vi "simulation.vi"(1 "Stop signaller":refnum<class "Signaller.lvclass">, 2 "Frequency refnum":refnum<vi>, 3 "Data input file refnum":refnum<vi>) -> ()   [LabVIEW 2015]
uses:
  Fit Parameters.ctl
  Physical Constants.ctl
  Internal Parameters.ctl
  System parameters.ctl
  Motor controller/Signaller/Signaller.lvclass
  <vilib>/Platform/TimedLoop/XDataNode/timing_clust.ctl
  <vilib>/Platform/TimedLoop/XDataNode/nitl_modes.ctl
  <vilib>/Platform/TimedLoop/XDataNode/wakeup.ctl
  <vilib>/Platform/TimedLoop/scheduler/LVUserAPI/_suppVIs/Create_1kHz_TSource.vi
  <vilib>/Utility/file.llb/Write Delimited Spreadsheet (string).vi
  <vilib>/platform/TimedLoop/XDataNode/XDataNode.xnode
  <vilib>/Platform/TimedLoop/XDataNode/XDNodeRunTimeDep.lvlib
panel:
  in  "Precision":i32=100 min=1
  in  "Reset simulation":bool
  in  "Paused":bool=TRUE
  out "Current time (simulated)":timestamp format="%<%H:%M:%S\n%B %d, %Y>T"
  in  "Stop simulation":bool
  in  "Data output file":path
  out "Polarization":dbl
  in  "Beam on":bool
  in  "Time per second (s)":dbl=1.0
  out "Seconds until next data":u32
  in  "# Sweeps":u32=250
  out "Fit parameters chooser":refnum<vi>
  in  "Sweep error":dbl=0.01 min=0.0 format="%#_13g"
  out "Start time":timestamp
  out "Polarization (unfuzzed)":dbl
  in  "Thermal fluctuations":dbl=0.01 min=0.0
  out "Pn (noisy)":dbl
  in  "System parameters":T1={"Frequency"=140.2, "System temperature"=1.0, "Beam current"=100.0}
  out "Internal parameters":T2={"Pe"=-1.0, "Pn"=0.0, "Alpha"=0.0, "Beta"=0.0, "C"=0.000136073, "Phi"=0.0, "Pe0"=-1.0, "Dose"=0.0, "Temperature"=1.0}
  in  "Physical constants":T3={"T1e (s)"=0.03, "T1n (s)"=1500.0}
  in  "Fit parameters":T4={"A"=0.572086, "S"=0.0835606, "M1"=140.286, "M2"=140.486}
  in  "Launch fit parameters chooser":bool
  out "Elapsed time (s)":dbl
  in  "Add 30 minutes":bool
  in  "30 minutes":bool
  in  "15 minutes":bool
  in  "5 minutes":bool
  in  "Time scale (min)":i64=5 min=1
  out "Polarization vs time":cluster{timestamp[], dbl[]}(graph)
  # "Advanced data and controls"
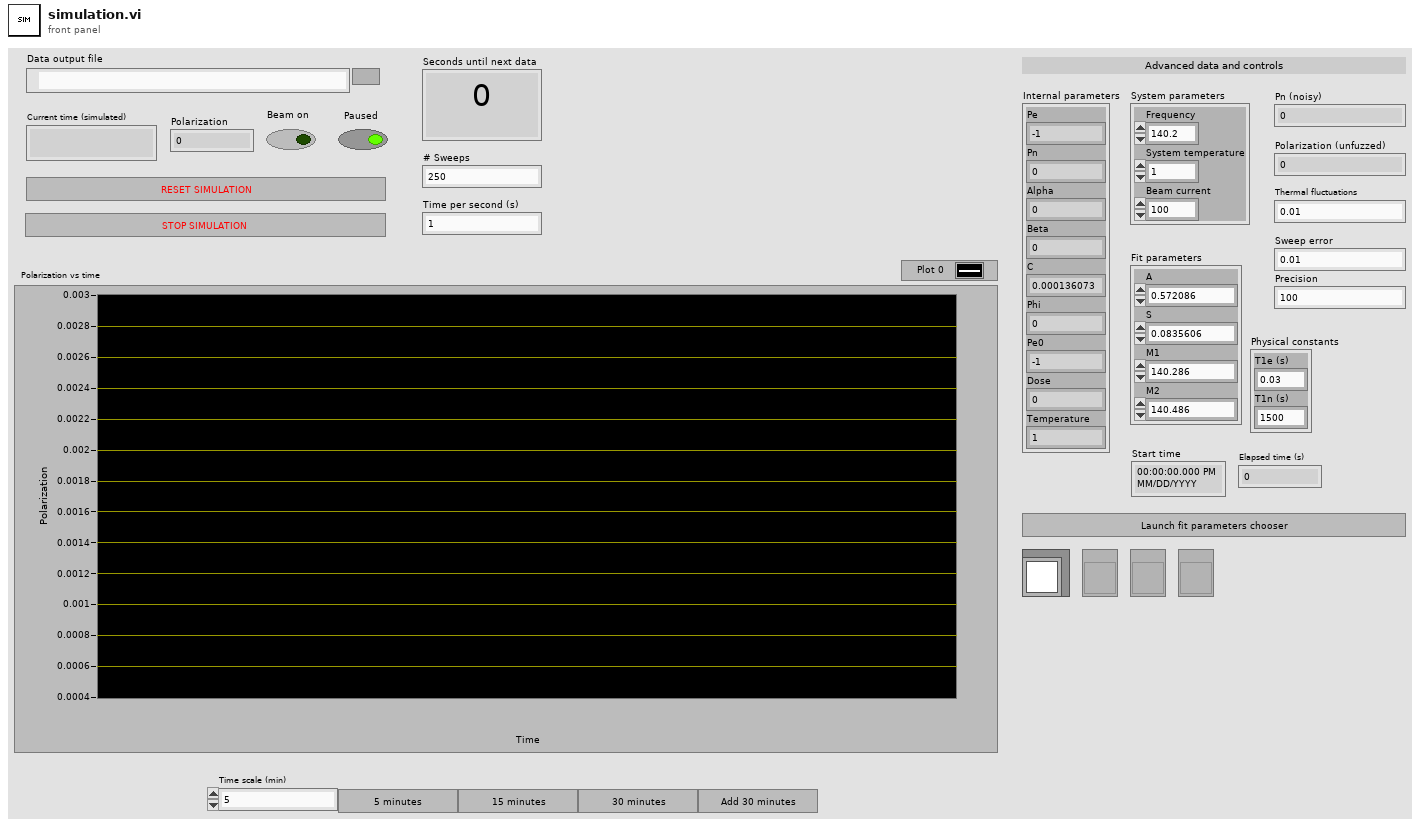
[diagram p1: front panel]
types:
  T1 = typedef "System parameters.ctl" = cluster{"Frequency":dbl, "System temperature":dbl, "Beam current":dbl}
  T2 = typedef "Internal Parameters.ctl" = cluster{"Pe":dbl, "Pn":dbl, "Alpha":dbl, "Beta":dbl, "C":dbl, "Phi":dbl, "Pe0":dbl, "Dose":dbl, "Temperature":dbl}
  T3 = typedef "Physical Constants.ctl" = cluster{"T1e (s)":dbl, "T1n (s)":dbl}
  T4 = typedef "Fit Parameters.ctl" = cluster{"A":dbl, "S":dbl, "M1":dbl, "M2":dbl}
  T5 = enum8{"Enabled", "Disabled", "Disabled and Grayed Out"}
  T6 = typedef "Semaphore RefNum" = refnum<k1>
  T7 = typedef "XDNodeRunTimeDep.lvlib/timing_clust.ctl" = cluster{"Expected End [f-1]":u64, "Actual End [f-1]":u64, "Finished Late? [f-1]":bool, "Expected End [i-1]":u64, "Actual End [i-1]":u64, "Finished Late? [i-1]":bool, "Expected Start [i]":u64, "Actual Start [i]":u64, "Expected Start [f]":u64, "Actual Start [f]":u64, "Source Name":string, "Structure Name":string, "Period":i64, "Deadline":i64, "Offset":i64, "Start":i64, "Priority":i32, "Timeout":i32, "Mode":T8, "Wakeup Reason":T9, "Error":errorcluster, "Source Type":string, "Secondary Source Type":string, "Global End Time":u64, "Global Start Time":u64, "Frame Duration":u64, "Iteration Duration":u64, "Assigned CPU":i32, "I/O Scan Engine Mode":u32}
  T8 = typedef "XDNodeRunTimeDep.lvlib/nitl_modes.ctl" = enum32{"No Change", "Process missed periods, maintain original phase", "Discard missed periods, maintain original phase", "Process missed periods, ignore original phase", "Discard missed periods, ignore original phase"}
  T9 = typedef "XDNodeRunTimeDep.lvlib/wakeup.ctl" = enum32{"Normal", "Aborted", "Asynchronous wakeup", "Timing source error", "Timed loop error", "Timeout"}
  T10 = typedef "internal_parameters.ctl" = cluster{"Pe":dbl, "Pn":dbl, "Alpha":dbl, "Beta":dbl, "C":dbl, "Phi":dbl, "Pe0":dbl, "Dose":dbl, "Temperature":dbl}
  T11 = typedef "LVRangeTypeDef.ctl" = cluster{"Minimum":dbl, "Maximum":dbl, "Increment":dbl, "Minor Increment":dbl, "Start":dbl}
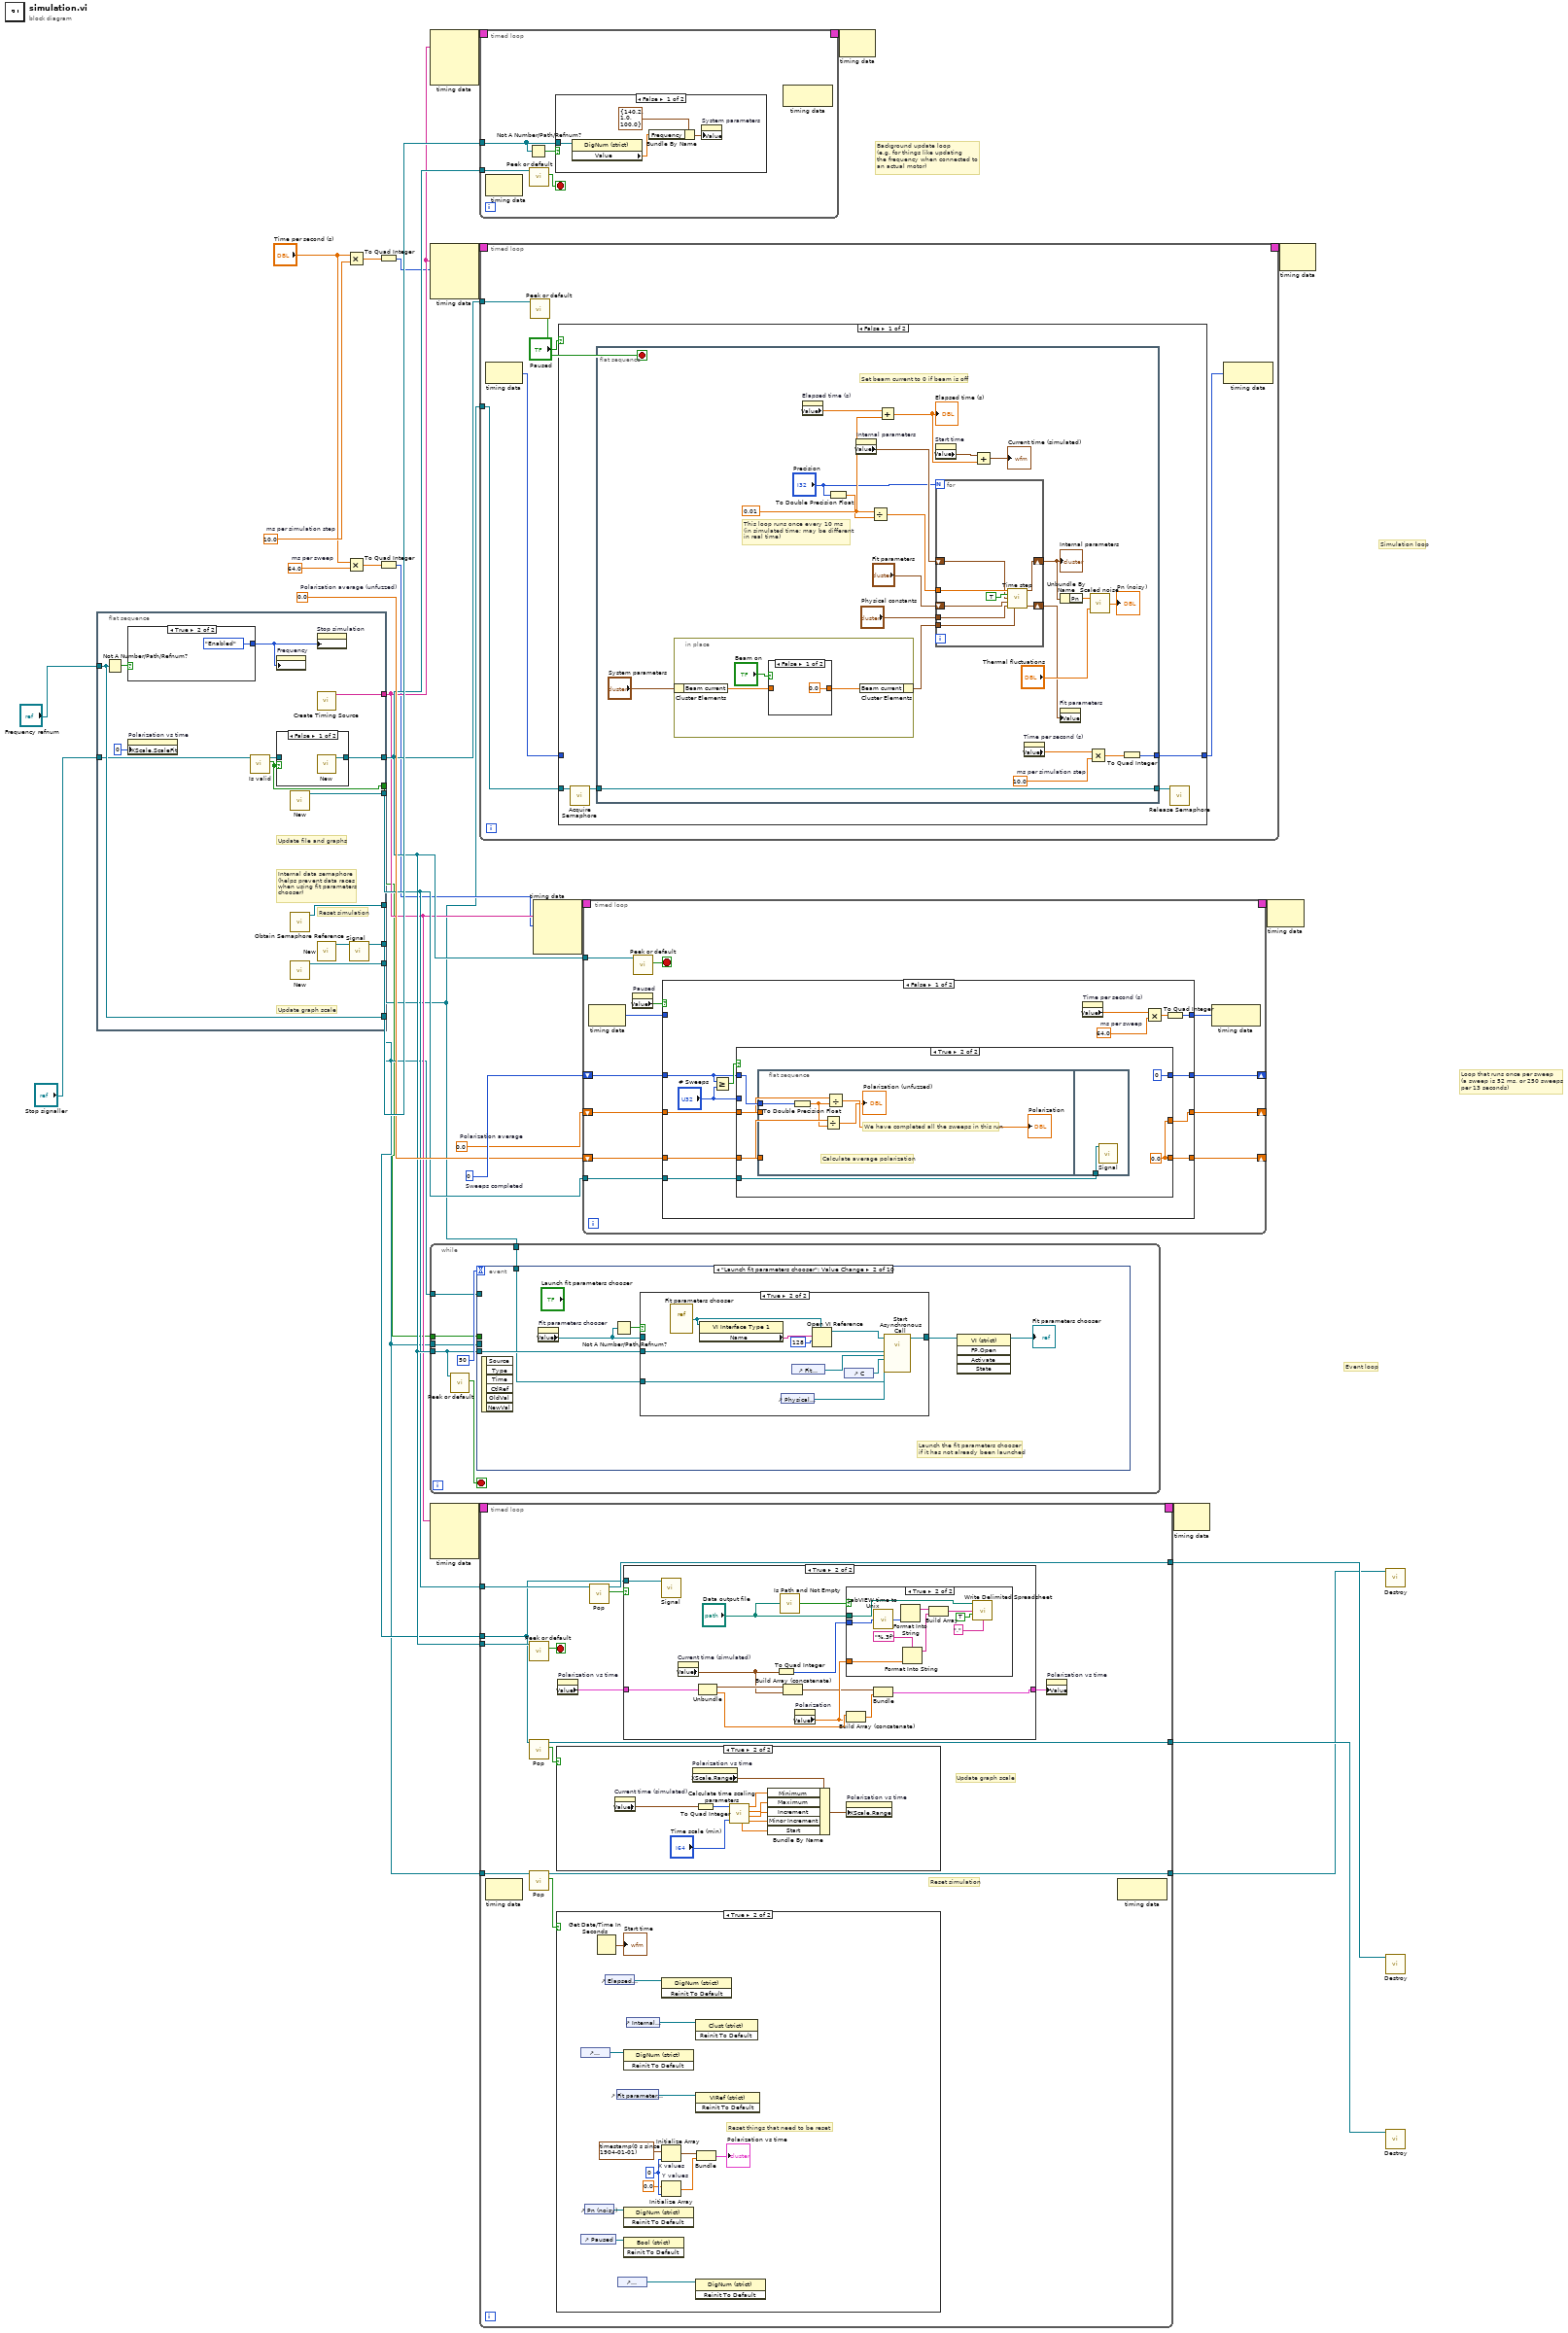
[diagram p0: block diagram]
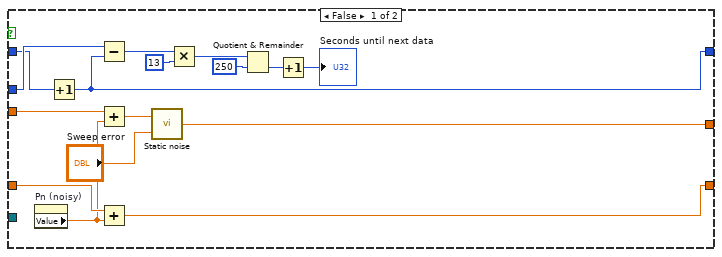
[diagram p6: hidden frame]
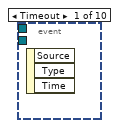
[diagram p11: hidden frame]
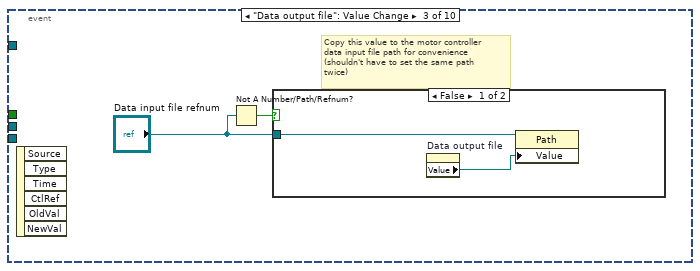
[diagram p13: hidden frame]
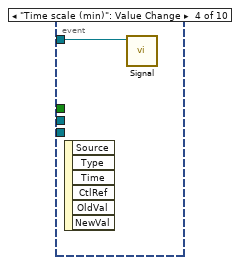
[diagram p15: hidden frame]
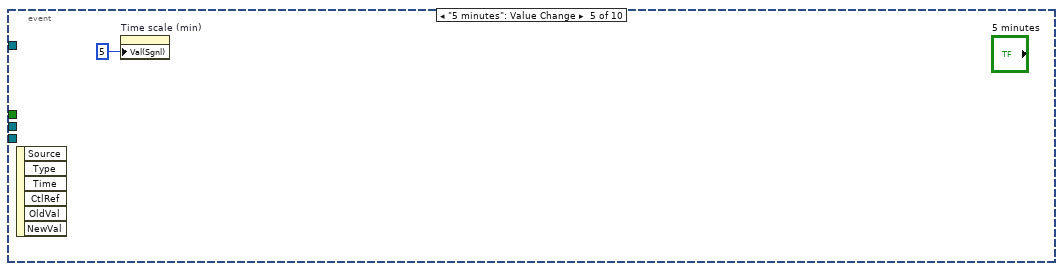
[diagram p16: hidden frame]
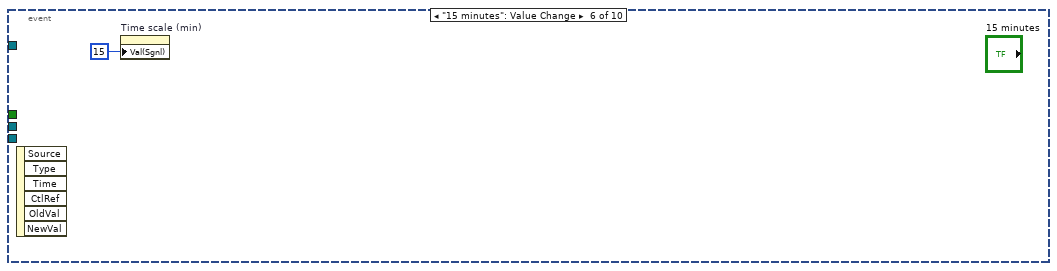
[diagram p17: hidden frame]
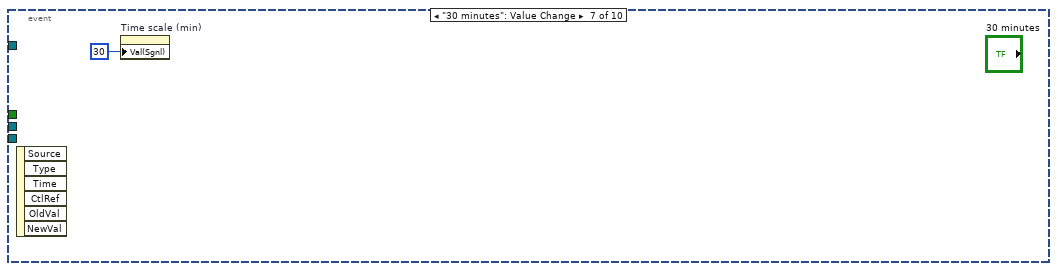
[diagram p18: hidden frame]
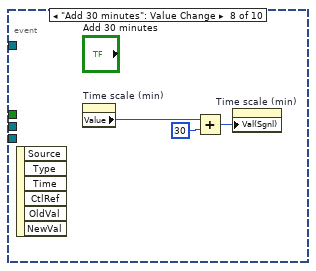
[diagram p19: hidden frame]
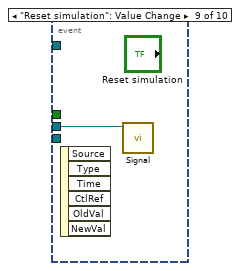
[diagram p20: hidden frame]
diagram:
  w6 = 64.0  # ms per sweep
  w10 = 10.0  # ms per simulation step
  w21 = 0.0  # Polarization average (unfuzzed)
  w22 = 0.0  # Polarization average
  w23 = u32 0  # Sweeps completed
  # "Loop that runs once per sweep\n(a sweep is 52 ms, or 250 sweeps\nper 13 seconds)"
  # "Background update loop\n(e.g. for things like updating\nthe frequency when connected to\nan actual motor)"
  # "Event loop"
  # "Simulation loop"
  n1 = flat-sequence {
    tunnel: "Frequency refnum" -> [w44]
    tunnel: [w36] -> w20
    tunnel: [w44] -> w30
    tunnel: [w41] -> w18
    tunnel: [w40] -> w12
    tunnel: "Stop signaller" -> [w38]
    tunnel: [w39] -> w13
    tunnel: [w35] -> w11
    tunnel: [w33] -> w2
    tunnel: [w32] -> w1
    frame #0 {
      # "Internal data semaphore\n(helps prevent data races\nwhen using fit parameters\nchooser)"
      # "Reset simulation"
      # "Update graph scale"
      # "Update file and graphs"
      n2 = Not A Number/Path/Refnum?(number/path/refnum=w44) -> (NaN/Path/Refnum?=w45:bool)
      n3 = case shown="True" w45 {
        tunnel: [T5."Disabled and Grayed Out" ("Disabled") T5."Enabled" ("Disabled")] -> w42
        frame False {
        }
        frame True {
        }
      }
      n4 = property on="Polarization vs time" class="XYGraph (strict)"("XScale.ScaleFit"=u8 0 ("X Scale.Scale Fit")) -> ()  [unwired: 2 in, 2 out]
      n5 = call "Is valid.vi"("Signaller in"=w38) -> ("Is valid?"=w35:bool, "Signaller out"=w37:refnum<class "Signaller.lvclass">)  [unwired: 8 in, 1 out]
      n6 = property on="Frequency" class="DigNum (strict)"("DisabledEnum"=w42) -> ()  [unwired: 2 in, 2 out]
      n7 = case shown="False" w35 {
        tunnel: w37 -> [_ w47]
        tunnel: [w46 w47] -> w36
        frame False {
          n8 = call "New.vi"() -> ("Signaller out"=w46:refnum<class "Signaller.lvclass">)  [unwired: 11 in]
        }
        frame True {
        }
      }
      n9 = call "New.vi"() -> ("Signaller out"=w41:refnum<class "Signaller.lvclass">)  [unwired: 11 in]
      n10 = call <vilib>:"Obtain Semaphore Reference.vi"() -> ("semaphore"=w32:T6)  [unwired: 5 in, 2 out]
      n11 = call "New.vi"() -> ("Signaller out"=w40:refnum<class "Signaller.lvclass">)  [unwired: 11 in]
      n12 = property on="Stop simulation" class="Bool"("DisabledEnum"=w42) -> ()  [unwired: 2 in, 2 out]
      n13 = call-poly <vilib>:"Create Timing Source.vi"() -> ("name (out)"=w39:string)  [unwired: 10 in, 1 out]
      n14 = call "New.vi"() -> ("Signaller out"=w34:refnum<class "Signaller.lvclass">)  [unwired: 11 in]
      n15 = call "Signal.vi"("Signaller in"=w34) -> ("Signaller out"=w33:refnum<class "Signaller.lvclass">)  [unwired: 9 in, 1 out]
    }
  }
  n16 = Multiply(x="Time per second (s)", y=w10) -> (x*y=w9:dbl)
  n17 = Multiply(x="Time per second (s)", y=w6) -> (x*y=w5:dbl)
  n18 = To Quad Integer(1:w9) -> (0:w8:i64)
  n19 = To Quad Integer(1:w5) -> (0:w4:i64)
  n20 = node-c288(w13) -> (w27:T7)  [unwired: 3 in]
  n21 = node-c288(w13, w8) -> (w29:T7)  [unwired: 2 in]
  n22 = while {
    tunnel: w20 -> [w54]
    tunnel: w12 -> [w53]
    tunnel: w11 -> [w52]
    tunnel: w2 -> [w51]
    tunnel: w1 -> [w50]
    stop <- w56 stop-if-true
    n23 = call "Peek or default.vi"("Signaller in"=w54) -> ("Has signal?"=w56:bool)  [unwired: 8 in, 2 out]
    n24 = event shown="[1] \"Launch fit parameters chooser\": Value Change" {
      selector: _ -> [_ _ _ _ _ _ _ _ _ _]
      dyn-events: _ -> [_ _ _ _ _ _ _ _ _ _]
      timeout: 50 -> [_ _ _ _ _ _ _ _ _ _]
      tunnel: w54 -> [_ w62 _ _ _ _ _ _ _ w87]
      tunnel: w53 -> [_ _ _ w78 _ _ _ _ _ _]
      tunnel: w52 -> [_ _ _ _ _ _ _ _ _ w86]
      tunnel: w51 -> [_ _ _ _ _ _ _ _ w85 _]
      tunnel: w50 -> [_ w58 _ _ _ _ _ _ _ _]
      event Timeout {
        n25 = event-data() -> ()  [unwired: 1 in, 3 out]
      }
      event "Launch fit parameters chooser": Value Change {
        # "Launch the fit parameters chooser\nif it has not already been launched"
        n26 = event-data() -> ()  [unwired: 1 in, 6 out]
        n27 = property on="Fit parameters chooser" class="VIRef (strict)"() -> ("Value"=w60:refnum<vi>)  [unwired: 2 in, 2 out]
        n28 = Not A Number/Path/Refnum?(number/path/refnum=w60) -> (NaN/Path/Refnum?=w61:bool)
        n29 = case shown="True" w61 {
          tunnel: w62 -> [_ w68]
          tunnel: w60 -> [w63 _]
          tunnel: [w63 w69] -> w59
          tunnel: w58 -> [_ w64]
          frame False {
          }
          frame True {
            n30 = vi-ref "Fit parameters chooser.vi"() -> (w71:refnum<vi>)
            n31 = property class="VI Interface Type 1"(reference=w71) -> ("Name"=w70:string)  [unwired: 1 in, 2 out]
            n32 = control-ref of="Physical constants"() -> (w65:refnum<vi>)
            n33 = control-ref of="Fit parameters"() -> (w67:refnum<vi>)
            n34 = Open VI Reference(type specifier VI Refnum (for type only)=w71, vi path=w70, options=128) -> (vi reference=w73:refnum<vi>)  [unwired: 3 in, 1 out]
            n35 = control-ref of="C"() -> (w66:refnum<vi>)
            n36 = call-by-ref "Start Asynchronous Call"(reference=w73, "Stop signaller"=w68, "Fit parameters refnum"=w67, "C refnum"=w66, "Physical constants refnum"=w65, "Simulation parameters semaphore"=w64) -> (reference out=w69:refnum<vi>)  [unwired: 12 in, 1 out]
          }
        }
        n37 = invoke class="VI (strict)" method="FP.Open"(reference=w59) -> (reference out=→"Fit parameters chooser":refnum<vi>)  [unwired: 4 in, 4 out]
      }
      event "Data output file": Value Change {
        # "Copy this value to the motor controller\ndata input file path for convenience\n(shouldn't have to set the same path\ntwice)"
        n38 = event-data() -> ()  [unwired: 1 in, 6 out]
        n39 = Not A Number/Path/Refnum?(number/path/refnum="Data input file refnum") -> (NaN/Path/Refnum?=w75:bool)
        n40 = case shown="False" w75 {
          tunnel: "Data input file refnum" -> [w77 _]
          frame False {
            n41 = property on="Data output file" class="Path"() -> ("Value"=w76:path)  [unwired: 2 in, 2 out]
            n42 = property class="Path"(reference=w77, "Value"=w76) -> ()  [unwired: 1 in, 2 out]
          }
          frame True {
          }
        }
      }
      event "Time scale (min)": Value Change {
        n43 = event-data() -> ()  [unwired: 1 in, 6 out]
        n44 = call "Signal.vi"("Signaller in"=w78) -> ()  [unwired: 9 in, 2 out]
      }
      event "5 minutes": Value Change {
        n45 = event-data() -> ()  [unwired: 1 in, 6 out]
        n46 = property on="Time scale (min)" class="DigNum (strict)"("Val(Sgnl)"=i64 5 ("Value (Signaling)")) -> ()  [unwired: 2 in, 2 out]
      }
      event "15 minutes": Value Change {
        n47 = event-data() -> ()  [unwired: 1 in, 6 out]
        n48 = property on="Time scale (min)" class="DigNum (strict)"("Val(Sgnl)"=i64 15 ("Value (Signaling)")) -> ()  [unwired: 2 in, 2 out]
      }
      event "30 minutes": Value Change {
        n49 = event-data() -> ()  [unwired: 1 in, 6 out]
        n50 = property on="Time scale (min)" class="DigNum (strict)"("Val(Sgnl)"=i64 30 ("Value (Signaling)")) -> ()  [unwired: 2 in, 2 out]
      }
      event "Add 30 minutes": Value Change {
        n51 = event-data() -> ()  [unwired: 1 in, 6 out]
        n52 = property on="Time scale (min)" class="DigNum (strict)"() -> ("Value"=w84:i64)  [unwired: 2 in, 2 out]
        n53 = Add(x=w84, y=i64 30) -> (x+y=w82:i64)
        n54 = property on="Time scale (min)" class="DigNum (strict)"("Val(Sgnl)"=w82) -> ()  [unwired: 2 in, 2 out]
      }
      event "Reset simulation": Value Change {
        n55 = event-data() -> ()  [unwired: 1 in, 6 out]
        n56 = call "Signal.vi"("Signaller in"=w85) -> ()  [unwired: 9 in, 2 out]
      }
      event "Stop simulation": Value Change {
        n57 = event-data() -> ()  [unwired: 1 in, 6 out]
        n58 = case shown="False" w86 {
          tunnel: w87 -> [w88 _]
          frame False {
            n59 = call "Signal.vi"("Signaller in"=w88) -> ()  [unwired: 9 in, 2 out]
          }
          frame True {
          }
        }
      }
    }
  }
  n60 = node-c288(w13) -> (w17:T7)  [unwired: 3 in]
  n61 = timed-loop {
    tunnel: w30 -> [w91]
    tunnel: w20 -> [w89]
    timing: w27 -> [_]
    timing-out: [_] -> w26
    stop <- w90 stop-if-true
    n62 = node-c288() -> ()  [unwired: 1 in, 1 out]
    n63 = Not A Number/Path/Refnum?(number/path/refnum=w91) -> (NaN/Path/Refnum?=w92:bool)
    n64 = call "Peek or default.vi"("Signaller in"=w89) -> ("Has signal?"=w90:bool)  [unwired: 8 in, 2 out]
    n65 = case shown="False" w92 {
      tunnel: w91 -> [w98 _]
      frame False {
        n66 = property class="DigNum (strict)"(reference=w98) -> ("Value"=w95:dbl)  [unwired: 1 in, 2 out]
        n67 = Bundle By Name(cluster=T1 {"Frequency"=140.2, "System temperature"=1.0, "Beam current"=100.0} ("System parameters"), "Frequency"=w95) -> (w97:T1)
        n68 = property on="System parameters" class="Clust (strict)"("Value"=w97) -> ()  [unwired: 2 in, 2 out]
      }
      frame True {
      }
    }
    n69 = node-c288() -> ()  [unwired: 1 in, 1 out]
  }
  n70 = timed-loop {
    tunnel: w20 -> [w103]
    timing: w29 -> [_]
    timing-out: [_] -> w28
    tunnel: w1 -> [w99]
    stop <- w104 stop-if-true
    n71 = node-c288() -> (w100:i64)  [unwired: 1 in]
    n72 = call "Peek or default.vi"("Signaller in"=w103) -> ("Has signal?"=w104:bool)  [unwired: 8 in, 2 out]
    n73 = case shown="False" "Paused" {
      tunnel: [w108 w145] -> w102
      tunnel: w100 -> [_ w145]
      tunnel: w99 -> [w107 _]
      frame False {
        n74 = call <vilib>:"Acquire Semaphore.vi"("semaphore"=w107) -> ("semaphore out"=w106:T6)  [unwired: 4 in, 2 out]
        n75 = flat-sequence {
          tunnel: [w117] -> w108
          tunnel: w106 -> [w115]
          tunnel: [w115] -> w105
          frame #0 {
            w119 = 10.0  # ms per simulation step
            w112 = 0.01
            # "This loop runs once every 10 ms\n(in simulated time; may be different\nin real time)"
            # "Set beam current to 0 if beam is off"
            n76 = in-place {
              n77 = in-place-cluster #1("System parameters") -> ("Beam current"=w141:dbl)
              n78 = case shown="False" "Beam on" {
                tunnel: w141 -> [_ w144]
                tunnel: [0.0 ("Beam current (nA)") w144] -> w140
                frame False {
                }
                frame True {
                }
              }
              n79 = in-place-cluster #1("Beam current"=w140) -> (w124:T1)
            }
            n80 = property on="Elapsed time (s)" class="DigNum (strict)"() -> ("Value"=w131:dbl)  [unwired: 2 in, 2 out]
            n81 = To Double Precision Float(number="Precision") -> (double precision float=w111:dbl)
            n82 = property on="Internal parameters" class="Clust (strict)"() -> ("Value"=w113:T10)  [unwired: 2 in, 2 out]
            n83 = Divide(x=w112, y=w111) -> (x/y=w109:dbl)
            n84 = Add(x=w131, y=w112) -> (x+y=w121:dbl)
            "Elapsed time (s)" <- w121
            n85 = property on="Start time" class="AbsTime (strict)"() -> ("Value"=w122:timestamp)  [unwired: 2 in, 2 out]
            n86 = for {
              N: "Precision" -> [_]
              tunnel: "Physical constants" -> [w139]
              tunnel: w124 -> [w137]
              tunnel: w109 -> [w135]
              shift-right: [w134] -> w116
              shift-left: "Fit parameters" -> [w138]
              shift-right: [w133] -> w114
              shift-left: w113 -> [w132]
              n87 = call "Time step.vi"("Time (s)"=w135, "Microwave on"=TRUE, "Internal parameters in"=w132, "Fit parameters"=w138, "Physical constants"=w139, "System parameters"=w137) -> ("Internal parameters out"=w133:T2, "Fit parameters out"=w134:T4)  [unwired: 8 in]
            }
            "Internal parameters" <- w114
            n88 = Add(x=w122, y=w121) -> (x+y=→"Current time (simulated)":timestamp)
            n89 = property on="Time per second (s)" class="DigNum (strict)"() -> ("Value"=w118:dbl)  [unwired: 2 in, 2 out]
            n90 = property on="Fit parameters" class="Clust (strict)"("Value"=w116) -> ()  [unwired: 2 in, 2 out]
            n91 = Unbundle By Name(w114) -> ("Pn"=w129:dbl)
            n92 = Multiply(x=w118, y=w119) -> (x*y=w120:dbl)
            n93 = call "Scaled noise.vi"("Fraction"="Thermal fluctuations", "Input"=w129) -> ("Output with noise"=→"Pn (noisy)":dbl)
            n94 = To Quad Integer(1:w120) -> (0:w117:i64)
          }
        }
        n95 = call <vilib>:"Release Semaphore.vi"("semaphore"=w105) -> ()  [unwired: 5 in, 2 out]
      }
      frame True {
      }
    }
    n96 = node-c288(w102) -> ()  [unwired: 1 out]
  }
  n97 = timed-loop {
    tunnel: w20 -> [w161]
    tunnel: w18 -> [w160]
    tunnel: [w159] -> w19
    timing: w17 -> [_]
    timing-out: [_] -> w16
    tunnel: w12 -> [w156]
    tunnel: [w157] -> w15
    tunnel: w2 -> [w155]
    tunnel: [w153] -> w3
    stop <- w162 stop-if-true
    # "Update graph scale"
    # "Reset simulation"
    n98 = node-c288() -> ()  [unwired: 1 in, 1 out]
    n99 = call "Peek or default.vi"("Signaller in"=w161) -> ("Has signal?"=w162:bool)  [unwired: 8 in, 2 out]
    n100 = call "Pop.vi"("Signaller in"=w156) -> ("Has signal"=w158:bool, "Signaller out"=w157:refnum<class "Signaller.lvclass">)  [unwired: 8 in, 1 out]
    n101 = call "Pop.vi"("Signaller in"=w155) -> ("Has signal"=w154:bool, "Signaller out"=w153:refnum<class "Signaller.lvclass">)  [unwired: 8 in, 1 out]
    n102 = case shown="True" w158 {
      frame False {
      }
      frame True {
        n103 = property on="Current time (simulated)" class="AbsTime (strict)"() -> ("Value"=w178:timestamp)  [unwired: 2 in, 2 out]
        n104 = property on="Polarization vs time" class="XYGraph (strict)"() -> ("XScale.Range"=w181:T11)  [unwired: 2 in, 2 out]
        n105 = To Quad Integer(1:w178) -> (0:w180:i64)
        n106 = call "Calculate time scaling parameters.vi"("Time"=w180, "Time scale (minutes)"="Time scale (min)") -> ("Minimum"=w184:dbl, "Maximum"=w185:dbl, "Increment"=w186:dbl, "Minor increment"=w187:dbl, "Start"=w183:dbl)  [unwired: 1 in]
        n107 = Bundle By Name(cluster=w181, "Minimum"=w184, "Maximum"=w185, "Increment"=w186, "Minor Increment"=w187, "Start"=w183) -> (w182:T11)
        n108 = property on="Polarization vs time" class="XYGraph (strict)"("XScale.Range"=w182) -> ()  [unwired: 2 in, 2 out]
      }
    }
    n109 = case shown="True" w154 {
      frame False {
      }
      frame True {
        w167 = 0 ("dimension size")
        # "Reset things that need to be reset"
        n110 = control-ref of="Polarization"() -> (w174:refnum<vi>)
        n111 = control-ref of="Paused"() -> (w164:refnum<vi>)
        n112 = control-ref of="Pn (noisy)"() -> (w173:refnum<vi>)
        n113 = Get Date/Time In Seconds() -> (seconds since 1Jan1904=→"Start time":timestamp)
        n114 = control-ref of="Elapsed time (s)"() -> (w172:refnum<vi>)
        n115 = control-ref of="Fit parameters chooser"() -> (w177:refnum<vi>)
        n116 = control-ref of="Polarization (unfuzzed)"() -> (w175:refnum<vi>)
        n117 = invoke class="DigNum (strict)" method="Reinit To Default"(reference=w174) -> ()  [unwired: 2 in, 3 out]
        n118 = invoke class="DigNum (strict)" method="Reinit To Default"(reference=w173) -> ()  [unwired: 2 in, 3 out]
        n119 = invoke class="Bool (strict)" method="Reinit To Default"(reference=w164) -> ()  [unwired: 2 in, 3 out]
        n120 = control-ref of="Internal parameters"() -> (w171:refnum<vi>)
        n121 = invoke class="DigNum (strict)" method="Reinit To Default"(reference=w172) -> ()  [unwired: 2 in, 3 out]
        n122 = Initialize Array "X values"(timestamp(0 s since 1904-01-01), w167) -> (w168:timestamp[])
        n123 = Initialize Array "Y values"(0.0, w167) -> (w169:dbl[])
        n124 = invoke class="Clust (strict)" method="Reinit To Default"(reference=w171) -> ()  [unwired: 2 in, 3 out]
        n125 = invoke class="VIRef (strict)" method="Reinit To Default"(reference=w177) -> ()  [unwired: 2 in, 3 out]
        n126 = invoke class="DigNum (strict)" method="Reinit To Default"(reference=w175) -> ()  [unwired: 2 in, 3 out]
        n127 = Bundle(w168, w169) -> (→"Polarization vs time":cluster{timestamp[], dbl[]})  [unwired: 1 in]
      }
    }
    n128 = property on="Polarization vs time" class="XYGraph (strict)"() -> ("Value"=w151:cluster{timestamp[], dbl[]})  [unwired: 2 in, 2 out]
    n129 = call "Pop.vi"("Signaller in"=w160) -> ("Has signal"=w163:bool, "Signaller out"=w159:refnum<class "Signaller.lvclass">)  [unwired: 8 in, 1 out]
    n130 = case shown="True" w163 {
      tunnel: w151 -> [w190 w200]
      tunnel: [w190 w193] -> w152
      tunnel: w156 -> [_ w191]
      frame False {
      }
      frame True {
        n131 = call "Signal.vi"("Signaller in"=w191) -> ()  [unwired: 9 in, 2 out]
        n132 = property on="Current time (simulated)" class="AbsTime (strict)"() -> ("Value"=w192:timestamp)  [unwired: 2 in, 2 out]
        n133 = Unbundle(w200) -> (w199:timestamp[], w198:dbl[])
        n134 = To Quad Integer(1:w192) -> (0:w197:i64)
        n135 = call <vilib>:"Is Path and Not Empty.vi"("path"="Data output file") -> ("Is Path and Not Empty?"=w202:bool)  [unwired: 4 in]
        n136 = Build Array (concatenate)(w199, w192) -> (w194:timestamp[])
        n137 = property on="Polarization" class="DigNum (strict)"() -> ("Value"=w196:dbl)  [unwired: 2 in, 2 out]
        n138 = case shown="True" w202 {
          tunnel: "Data output file" -> [_ w209]
          tunnel: w197 -> [_ w208]
          tunnel: w196 -> [_ w205]
          frame False {
          }
          frame True {
            n139 = call "LabVIEW time to Unix.vi"("LabVIEW time"=w208) -> ("Unix time"=w207:i64)
            n140 = Format Into String(w207) -> (resulting string=w206:string)  [unwired: 3 in, 1 out]
            n141 = Format Into String(format string="%.3f", w205) -> (resulting string=w203:string)  [unwired: 2 in, 1 out]
            n142 = Build Array(w206, w203) -> (w210:string[])
            n143 = call-poly <vilib>:"Write Delimited Spreadsheet.vi"("file path (dialog if empty)"=w209, "1D data"=w210, "append to file? (F)"=TRUE, "delimiter (\\t)"="," ("delimiter (\\t)")) -> ()  [unwired: 10 in, 2 out]
          }
        }
        n144 = Build Array (concatenate)(w198, w196) -> (w195:dbl[])
        n145 = Bundle(w194, w195) -> (w193:cluster{timestamp[], dbl[]})  [unwired: 1 in]
      }
    }
    n146 = property on="Polarization vs time" class="XYGraph (strict)"("Value"=w152) -> ()  [unwired: 2 in, 2 out]
    n147 = node-c288() -> ()  [unwired: 1 in, 1 out]
  }
  n148 = node-c288(w13, w4) -> (w25:T7)  [unwired: 2 in]
  n149 = timed-loop {
    timing: w25 -> [_]
    timing-out: [_] -> w24
    tunnel: w20 -> [w223]
    shift-right: [w221] -> _
    shift-left: w23 -> [w222]
    shift-right: [w219] -> _
    shift-left: w22 -> [w220]
    shift-right: [w217] -> _
    shift-left: w21 -> [w218]
    tunnel: w18 -> [w216]
    stop <- w224 stop-if-true
    n150 = node-c288() -> (w213:i64)  [unwired: 1 in]
    n151 = property on="Paused" class="Bool (strict)"() -> ("Value"=w214:bool)  [unwired: 2 in, 2 out]
    n152 = call "Peek or default.vi"("Signaller in"=w223) -> ("Has signal?"=w224:bool)  [unwired: 8 in, 2 out]
    n153 = case shown="False" w214 {
      tunnel: w222 -> [w236 w270]
      tunnel: [w235 w270] -> w221
      tunnel: w220 -> [w233 w269]
      tunnel: [w232 w269] -> w219
      tunnel: w218 -> [w231 w268]
      tunnel: [w230 w268] -> w217
      tunnel: w216 -> [w229 _]
      tunnel: [w226 w267] -> w215
      tunnel: w213 -> [_ w267]
      frame False {
        w228 = 64.0  # ms per sweep
        n154 = Greater Or Equal?(x=w236, y="# Sweeps") -> (x >= y?=w237:bool)
        n155 = case shown="True" w237 {
          tunnel: w236 -> [w252 w257]
          tunnel: [w251 u32 0] -> w235
          tunnel: "# Sweeps" -> [w253 _]
          tunnel: w233 -> [w244 w258]
          tunnel: [w242 w255] -> w232
          tunnel: w231 -> [w240 w256]
          tunnel: [w238 w255] -> w230
          tunnel: w229 -> [_ w254]
          frame False {
            n156 = property on="Pn (noisy)" class="DigNum (strict)"() -> ("Value"=w239:dbl)  [unwired: 2 in, 2 out]
            n157 = Increment(x=w252) -> (x+1=w251:u32)
            n158 = Subtract(x=w253, y=w251) -> (x-y=w250:u32)
            n159 = Add(x=w244, y=w239) -> (x+y=w243:dbl)
            n160 = Add(x=w240, y=w239) -> (x+y=w238:dbl)
            n161 = call "Static noise.vi"("Fraction"="Sweep error", "Input"=w243) -> ("Output with noise"=w242:dbl)
            n162 = Multiply(x=w250, y=u32 13) -> (x*y=w248:u32)
            n163 = Quotient & Remainder(x=w248, y=u32 250) -> (floor(x/y)=w246:u32)  [unwired: 1 out]
            n164 = Increment(x=w246) -> (x+1=→"Seconds until next data":u32)
          }
          frame True {
            w255 = 0.0
            n165 = flat-sequence {
              tunnel: w258 -> [w265]
              tunnel: w257 -> [w264]
              tunnel: w256 -> [w262]
              tunnel: w254 -> [w266]
              frame #0 {
                # "Calculate average polarization"
                # "We have completed all the sweeps in this run"
                n166 = To Double Precision Float(number=w264) -> (double precision float=w261:dbl)
                n167 = Divide(x=w262, y=w261) -> (x/y=→"Polarization (unfuzzed)":dbl)
                n168 = Divide(x=w265, y=w261) -> (x/y=→"Polarization":dbl)
              }
              frame #1 {
                n169 = call "Signal.vi"("Signaller in"=w266) -> ()  [unwired: 9 in, 2 out]
              }
            }
          }
        }
        n170 = property on="Time per second (s)" class="DigNum (strict)"() -> ("Value"=w227:dbl)  [unwired: 2 in, 2 out]
        n171 = Multiply(x=w227, y=w228) -> (x*y=w225:dbl)
        n172 = To Quad Integer(1:w225) -> (0:w226:i64)
      }
      frame True {
      }
    }
    n173 = node-c288(w215) -> ()  [unwired: 1 out]
  }
  n174 = node-c288(w26) -> ()  [unwired: 1 out]
  n175 = node-c288(w16) -> ()  [unwired: 1 out]
  n176 = node-c288(w24) -> ()  [unwired: 1 out]
  n177 = node-c288(w28) -> ()  [unwired: 1 out]
  n178 = call "Destroy.vi"("Signaller in"=w3) -> ()  [unwired: 10 in, 1 out]
  n179 = call "Destroy.vi"("Signaller in"=w19) -> ()  [unwired: 10 in, 1 out]
  n180 = call "Destroy.vi"("Signaller in"=w15) -> ()  [unwired: 10 in, 1 out]
